vi "About.vi"(8 "error in (no error)":errorcluster) -> (0 "error out":errorcluster)   [LabVIEW 2012]
panel:
  in  "OK Button":bool
  in  "Tab Control":enum32{"About HeFTy", "About Patents"}(tab)
  out "License Information":string
  # "HeFTy"
  # "v 1.8.0"
  # "January 29, 2014"
  # "Copyright 2014, Richard A. Ketchum and Apatite to Zircon, Inc."
  # "Dpar is protected by U.S. Patent 5,267,274 and Australian Patent 658,800, both owned by Raymond A. Donelick.\n\nLicense to use Dpar is hereby granted to all academic institutions for purposes of not-for-profit research for not-for-profit entities. \n\nAll other use of Dpar is prohibited  without written permission of Raymond A. Donelick."
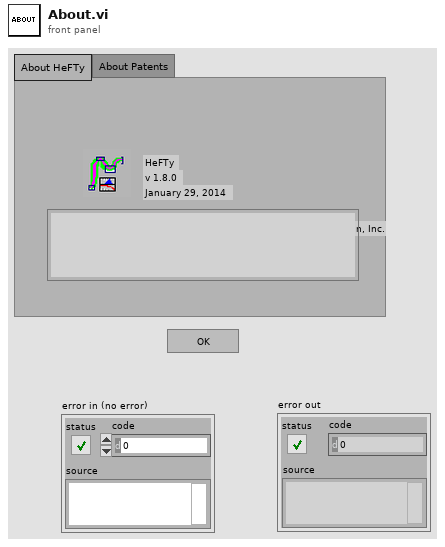
[diagram p1: front panel]
types:
  T1 = enum32{"Default", "TOTAL_DEMO", "EXXON_MOBIL_LIC", "ANDARKO_LIC", "STATOIL_LIC", "APT", "PB"}
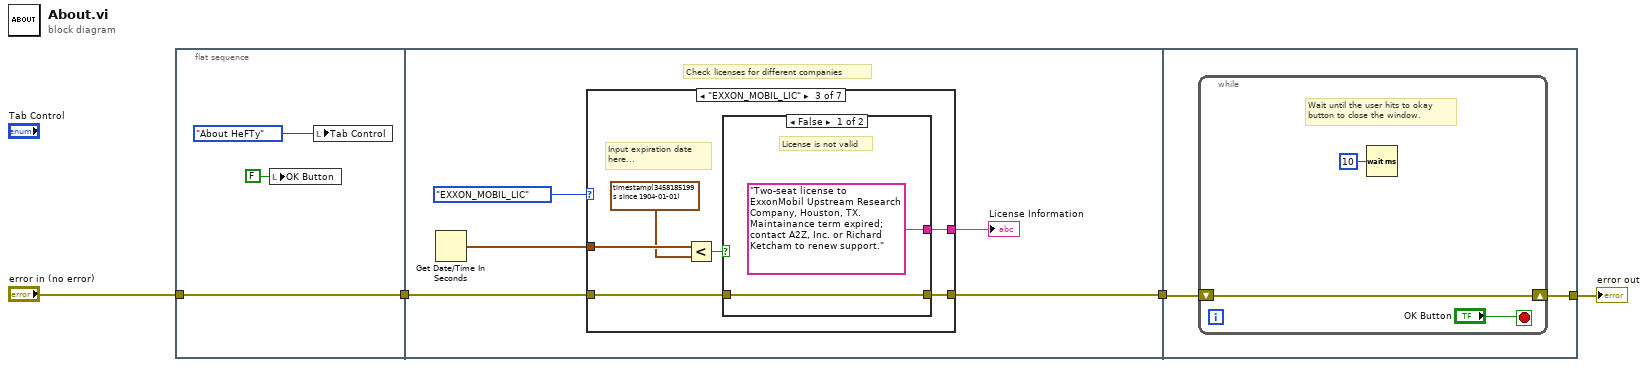
[diagram p0: block diagram]
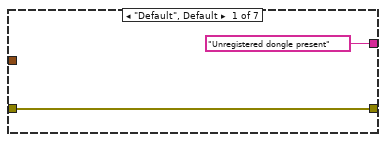
[diagram p2: hidden frame]
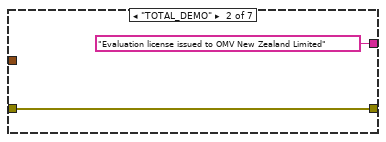
[diagram p3: hidden frame]
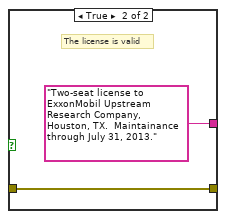
[diagram p4: hidden frame]
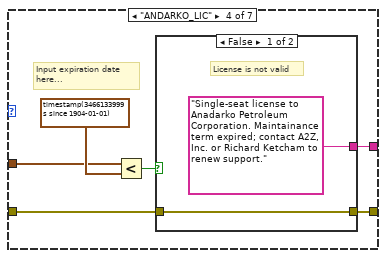
[diagram p5: hidden frame]
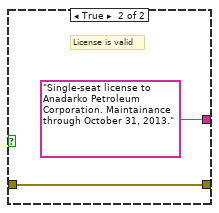
[diagram p6: hidden frame]
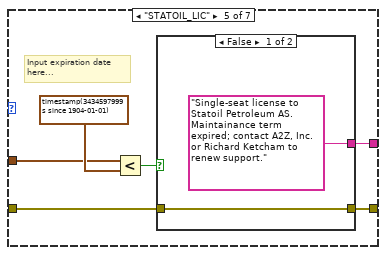
[diagram p7: hidden frame]
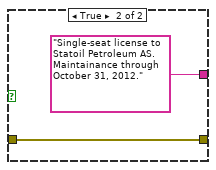
[diagram p8: hidden frame]
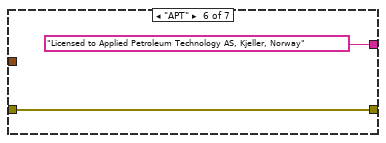
[diagram p9: hidden frame]
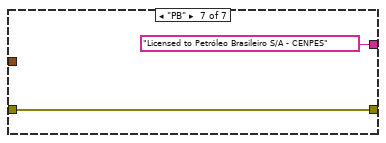
[diagram p10: hidden frame]
diagram:
  n1 = flat-sequence {
    tunnel: "error in (no error)" -> [w6]
    tunnel: [w6] -> w2
    tunnel: w2 -> [w12]
    tunnel: [w10] -> w1
    tunnel: [w52] -> w3
    tunnel: w1 -> [w51]
    frame #0 {
      n2 = local write "OK Button"(FALSE ("OK Button")) -> ()
      n3 = local write "Tab Control"(enum32{"About HeFTy", "About Patents"}."About HeFTy" ("Tab Control")) -> ()
    }
    frame #1 {
      # "Check licenses for different companies"
      n4 = Get Date/Time In Seconds() -> (seconds since 1Jan1904=w8:timestamp)
      n5 = case shown="\"EXXON_MOBIL_LIC\"" T1."EXXON_MOBIL_LIC" {
        tunnel: w12 -> [w14 w16 w20 w29 w39 w47 w50]
        tunnel: [w14 w16 w19 w28 w38 w47 w50] -> w10
        tunnel: ["Unregistered dongle present" "Evaluation license issued to OMV New Zealand Limited" w17 w27 w37 "Licensed to Applied Petroleum Technology AS, Kjeller, Norway" "Licensed to Petróleo Brasileiro S/A - CENPES"] -> w9
        tunnel: w8 -> [_ _ w22 w31 w41 _ _]
        frame "Default", Default {
        }
        frame "TOTAL_DEMO" {
        }
        frame "EXXON_MOBIL_LIC" {
          # "Input expiration date\nhere..."
          n6 = Less?(x=w22, y=timestamp(3458185199 s since 1904-01-01)) -> (x < y?=w21:bool)
          n7 = case shown="False" w21 {
            tunnel: w20 -> [w24 w26]
            tunnel: [w24 w26] -> w19
            tunnel: ["Two-seat license to ExxonMobil Upstream Research Company, Houston, TX.  Maintainance term expired; contact A2Z, Inc. or Richard Ketcham to renew support." "Two-seat license to ExxonMobil Upstream Research Company, Houston, TX.  Maintainance through July 31, 2013."] -> w17
            frame False {
              # "License is not valid"
            }
            frame True {
              # "The license is valid"
            }
          }
        }
        frame "ANDARKO_LIC" {
          # "Input expiration date\nhere..."
          n8 = Less?(x=w31, y=timestamp(3466133999 s since 1904-01-01)) -> (x < y?=w30:bool)
          n9 = case shown="False" w30 {
            tunnel: w29 -> [w33 w36]
            tunnel: [w33 w36] -> w28
            tunnel: ["Single-seat license to Anadarko Petroleum Corporation. Maintainance term expired; contact A2Z, Inc. or Richard Ketcham to renew support." "Single-seat license to Anadarko Petroleum Corporation. Maintainance through October 31, 2013."] -> w27
            frame False {
              # "License is not valid"
            }
            frame True {
              # "License is valid"
            }
          }
        }
        frame "STATOIL_LIC" {
          # "Input expiration date\nhere..."
          n10 = Less?(x=w41, y=timestamp(3434597999 s since 1904-01-01)) -> (x < y?=w40:bool)
          n11 = case shown="False" w40 {
            tunnel: w39 -> [w44 w46]
            tunnel: [w44 w46] -> w38
            tunnel: ["Single-seat license to Statoil Petroleum AS.  Maintainance term expired; contact A2Z, Inc. or Richard Ketcham to renew support." "Single-seat license to Statoil Petroleum AS.  Maintainance through October 31, 2012."] -> w37
            frame False {
            }
            frame True {
            }
          }
        }
        frame "APT" {
        }
        frame "PB" {
        }
      }
      "License Information" <- w9
    }
    frame #2 {
      n12 = while {
        shift-right: [w55] -> w52
        shift-left: w51 -> [w55]
        stop <- "OK Button" stop-if-true
        # "Wait until the user hits to okay\nbutton to close the window."
        n13 = Wait (ms)(milliseconds to wait=u32 10) -> ()  [unwired: 1 out]
      }
    }
  }
  "error out" <- w3
